vi "AMZ_S3_APIHLP_Set MFA Header.vi"(8 "error in (no error)":errorcluster, 10 "Auth device data":T2, 11 "HTTP Headers in":T1[](array[typedef])) -> (0 "error out":errorcluster, 2 "Header set?":bool, 3 "HTTP Headers":T1[](array[typedef]))   [LabVIEW 2015, in "LV Interface for Amazon S3.lvlib"]
uses:
  LV Interface for Amazon S3.lvlib
  Typedefs/AMZ_S3_Auth Device Data.ctl
  Typedefs/AMZ_S3_HTTP Header-Value pair.ctl
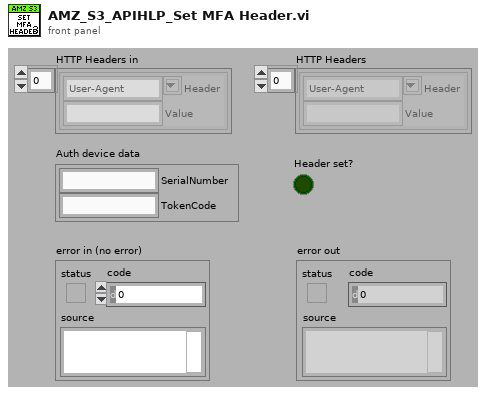
[diagram p1: front panel]
types:
  T1 = typedef "LV Interface for Amazon S3.lvlib/AMZ_S3_HTTP Header-Value pair.ctl" = cluster{"Header":string, "Value":string}
  T2 = typedef "LV Interface for Amazon S3.lvlib/AMZ_S3_Auth Device Data.ctl" = cluster{"SerialNumber":string, "TokenCode":string}
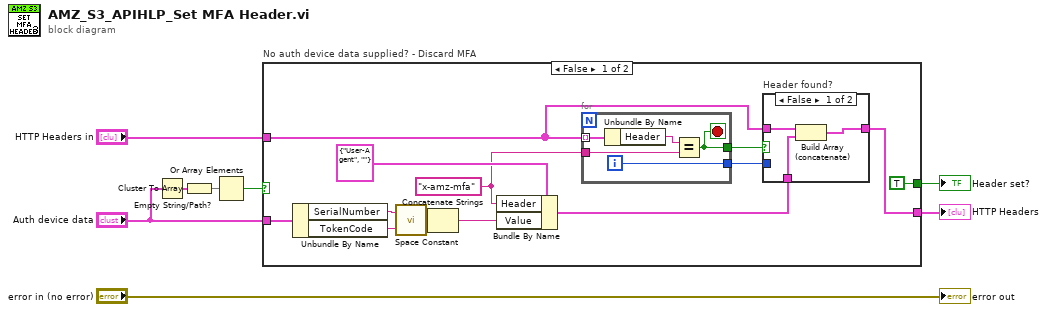
[diagram p0: block diagram]
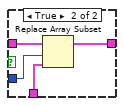
[diagram p2: hidden frame]
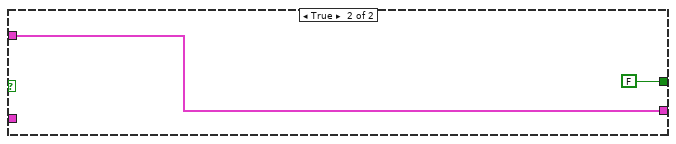
[diagram p3: hidden frame]
diagram:
  n1 = Empty String/Path?(string/path="Auth device data") -> (empty?=w8:cluster{"SerialNumber":bool, "TokenCode":bool})
  n2 = Cluster To Array(cluster=w8) -> (array=w7:bool[])
  n3 = Or Array Elements(Boolean array=w7) -> (logical OR=w2:bool)
  n4 = case "No auth device data supplied? - Discard MFA" shown="False" w2 {
    tunnel: "Auth device data" -> [w21 _]
    tunnel: [w10 w35] -> w4
    tunnel: "HTTP Headers in" -> [w12 w35]
    tunnel: [TRUE FALSE] -> w1
    frame False {
      w15 = "x-amz-mfa" ("Header")
      n5 = Unbundle By Name(w21) -> ("SerialNumber"=w20:string, "TokenCode"=w19:string)
      n6 = call <vilib>:"Space Constant.vi"() -> ("String"=w18:string)
      n7 = Concatenate Strings(w20, w18, w19) -> (w16:string)
      n8 = Bundle By Name(cluster=T1 {"Header"="User-Agent", "Value"=""} ("HTTP Header-Value pair"), "Header"=w15, "Value"=w16) -> (w11:T1)
      n9 = for {
        tunnel: w12 -> [w33] mode=indexing
        tunnel: w15 -> [w31]
        tunnel: [w30] -> w14
        tunnel: [w29] -> w13
        i -> [w29]
        stop <- w30 stop-if-true
        n10 = Unbundle By Name(w33) -> ("Header"=w32:string)
        n11 = Equal?(x=w32, y=w31) -> (x = y?=w30:bool)
      }
      n12 = case "Header found?" shown="False" w14 {
        tunnel: w13 -> [_ w27]
        tunnel: w12 -> [w24 w28]
        tunnel: w11 -> [w22 w26]
        tunnel: [w23 w25] -> w10
        frame False {
          n13 = Build Array (concatenate)(w24, w22) -> (w23:T1[])
        }
        frame True {
          n14 = Replace Array Subset(array=w28, new element=w26, index=w27) -> (w25:T1[])
        }
      }
    }
    frame True {
    }
  }
  "HTTP Headers" <- w4
  "Header set?" <- w1
  "error out" <- "error in (no error)"
